vi "Target4.vi"() -> ()   [LabVIEW 2025]
uses:
  <vilib>/Platform/TimedLoop/XDataNode/timing_clust.ctl
  <vilib>/Platform/TimedLoop/XDataNode/nitl_modes.ctl
  <vilib>/Platform/TimedLoop/XDataNode/wakeup.ctl
  <vilib>/rvi/Emulation/niFpgaSctlEmulationGetInTimedLoop.vi
  <vilib>/rvi/Emulation/niFpgaEmulationReportErrorSimple.vi
  <vilib>/rvi/Emulation/niFpgaGetClockAttributes.vi
  <vilib>/rvi/Emulation/niFpgaCriticalErrorInLSC.vi
  <vilib>/rvi/linearAlgebra/MatrixMultiply/simVIs/SubVI/nifxpla_MatrixMultiply_SimMatrixSizes.vi
  <vilib>/rvi/linearAlgebra/MatrixMultiply/simVIs/SubVI/nifxpla_MatrixMultiply_Sim4WireAdapterVector.vi
  <vilib>/rvi/linearAlgebra/MatrixMultiply/simVIs/SubVI/nifxpla_MatrixMultiply_SimFrameHandShake.vi
  <vilib>/rvi/linearAlgebra/MatrixMultiply/simVIs/SubVI/nifxpla_MatrixMultiply_SimVectorDataBuffer.vi
  <vilib>/rvi/linearAlgebra/MatrixMultiply/simVIs/SubVI/nifxpla_MatrixMultiply_SimNestedIndex.vi
  <vilib>/rvi/ClientSDK/Core/DevComputerLib/Private/Multiply(dfxp64).vi
  <vilib>/rvi/ClientSDK/Core/DevComputerLib/Private/Dfxp128ToDfxp256.vi
  <vilib>/rvi/ClientSDK/Core/DevComputerLib/Private/Add(dfxp256).vi
  <vilib>/rvi/ClientSDK/Core/DevComputerLib/Private/Subtract(dfxp256).vi
  <vilib>/rvi/ClientSDK/Core/DevComputerLib/Private/ToDfxp64(dfxp256).vi
  <vilib>/eio/utilities/niEioResolveVilibRelativePath.vi
  <vilib>/rvi/interface/RandomDataEmulation/niFpgaRandomDataHandleErrors.vi
  <vilib>/platform/TimedLoop/XDataNode/XDataNode.xnode
  <vilib>/rvi/linearAlgebra/MatrixMultiply/XNode/nifxpla_MatrixMultiply.xnode
  <vilib>/rvi/linearAlgebra/MatrixMultiply/simVIs/nifxpla_MatrixMultiply_SimTemplateEinEout.vi
  <vilib>/rvi/linearAlgebra/MatrixMultiply/simVIs/nifxpla_MatrixMultiply_SimTemplateEinVout.vi
  <vilib>/rvi/linearAlgebra/MatrixMultiply/simVIs/nifxpla_MatrixMultiply_SimTemplateVinEout.vi
  <vilib>/rvi/linearAlgebra/MatrixMultiply/simVIs/nifxpla_MatrixMultiply_SimTemplateVinVout.vi
  <vilib>/rvi/DataTransferAndStorage/Container/XNode/niFpgaContainer.xnode
  <vilib>/rvi/interface/RandomDataEmulation/nirviRandomDataFpgaReadWriteTemplate.vi
  <vilib>/Platform/TimedLoop/XDataNode/XDNodeRunTimeDep.lvlib
panel:
  out "operation overflow":bool
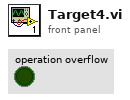
[diagram p1: front panel]
types:
  T1 = typedef "XDNodeRunTimeDep.lvlib/timing_clust.ctl" = cluster{"Expected End [f-1]":u64, "Actual End [f-1]":u64, "Finished Late? [f-1]":bool, "Expected End [i-1]":u64, "Actual End [i-1]":u64, "Finished Late? [i-1]":bool, "Expected Start [i]":u64, "Actual Start [i]":u64, "Expected Start [f]":u64, "Actual Start [f]":u64, "Source Name":string, "Structure Name":string, "Period":i64, "Deadline":i64, "Offset":i64, "Start":i64, "Priority":i32, "Timeout":i32, "Mode":T2, "Wakeup Reason":T3, "Error":errorcluster, "Source Type":string, "Secondary Source Type":string, "Global End Time":u64, "Global Start Time":u64, "Frame Duration":u64, "Iteration Duration":u64, "Assigned CPU":i32, "I/O Scan Engine Mode":u32}
  T2 = typedef "XDNodeRunTimeDep.lvlib/nitl_modes.ctl" = enum32{"No Change", "Process missed periods, maintain original phase", "Discard missed periods, maintain original phase", "Process missed periods, ignore original phase", "Discard missed periods, ignore original phase"}
  T3 = typedef "XDNodeRunTimeDep.lvlib/wakeup.ctl" = enum32{"Normal", "Aborted", "Asynchronous wakeup", "Timing source error", "Timed loop error", "Timeout"}
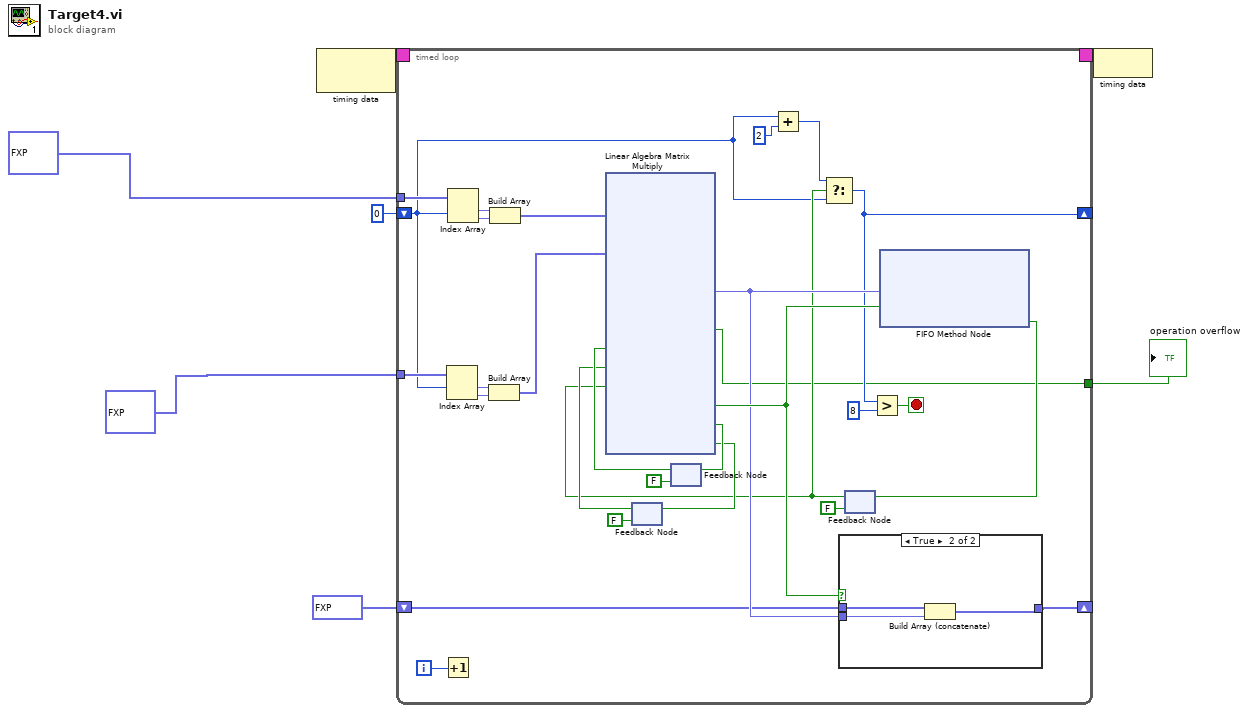
[diagram p0: block diagram]
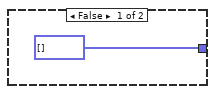
[diagram p2: hidden frame]
diagram:
  n1 = node-c288() -> (w7:T1)  [unwired: 1 in]
  n2 = timed-loop {
    timing: w7 -> [_]
    timing-out: [_] -> w6
    tunnel: fxp<+,1,2>[] [2.0, 2.0] -> [w36]
    tunnel: fxp<+,1,1>[] [1.0, 1.0] -> [w30]
    shift-right: [w12] -> _
    shift-left: 0 -> [w8]
    shift-right: [w20] -> _
    shift-left: fxp<+/-,64,35>[] [0.0, 0.0] ("cr") -> [w21]
    tunnel: [w9] -> w3
    i -> [w25]
    stop <- w13 stop-if-true
    n3 = Increment(x=w25) -> ()  [unwired: 1 out]
    n4 = Index Array(array=w30, index #1=w8) -> (element #1=w32:fxp<+,1,1>, element #2=w31:fxp<+,1,1>)  [unwired: 1 in]
    n5 = Index Array(array=w36, index #1=w8) -> (element #1=w35:fxp<+,1,2>, element #2=w34:fxp<+,1,2>)  [unwired: 1 in]
    n6 = Build Array(w32, w31) -> (w29:fxp<+,1,1>[])
    n7 = Build Array(w35, w34) -> (w33:fxp<+,1,2>[])
    n8 = feedback #1(FALSE ("ready for b")) -> (w24:bool)
    n9 = feedback #2(FALSE ("ready for a")) -> (w26:bool)
    n10 = Add(x=w8, y=2) -> (x+y=w15:i32)
    n11 = feedback #3(FALSE ("Ready for Input")) -> (w14:bool)
    n12 = xnode ("Linear Algebra Matrix Multiply")("ar"=w33, "br"=w29, "a valid"=w26, "b valid"=w24, "ready for output (T)"=w14) -> ("cr"=w22:fxp<+/-,32,16>, "operation overflow"=w9:bool, "output valid"=w23:bool, "ready for a"=w28:bool, "ready for b"=w27:bool)  [unwired: 2 in, 1 out]
    n13 = feedback-in #1(w27) -> ()
    n14 = feedback-in #2(w28) -> ()
    n15 = Select(t=w15, s=w14, f=w8) -> (s? t:f=w12:i32)
    n16 = case shown="True" w23 {
      tunnel: [fxp<+,1,1>[] [] w40] -> w20
      tunnel: w22 -> [_ w38]
      tunnel: w21 -> [_ w39]
      frame False {
      }
      frame True {
        n17 = Build Array (concatenate)(w39, w38) -> (w40:fxp<+/-,64,35>[])
      }
    }
    n18 = Greater?(x=w12, y=8) -> (0:w13:bool)
    n19 = xnode ("FIFO Method Node")("Element"=w22, "Input Valid"=w23) -> ("Ready for Input"=w18:bool)  [unwired: 1 in, 1 out]
    n20 = feedback-in #3(w18) -> ()
  }
  "operation overflow" <- w3
  n21 = node-c288(w6) -> ()
